vi "current viewer.vi"() -> ()   [LabVIEW 2018]
panel:
  out "Motor Current Versus Time":sgl[][](graph)
  in  "File":path
  # "v1.01"
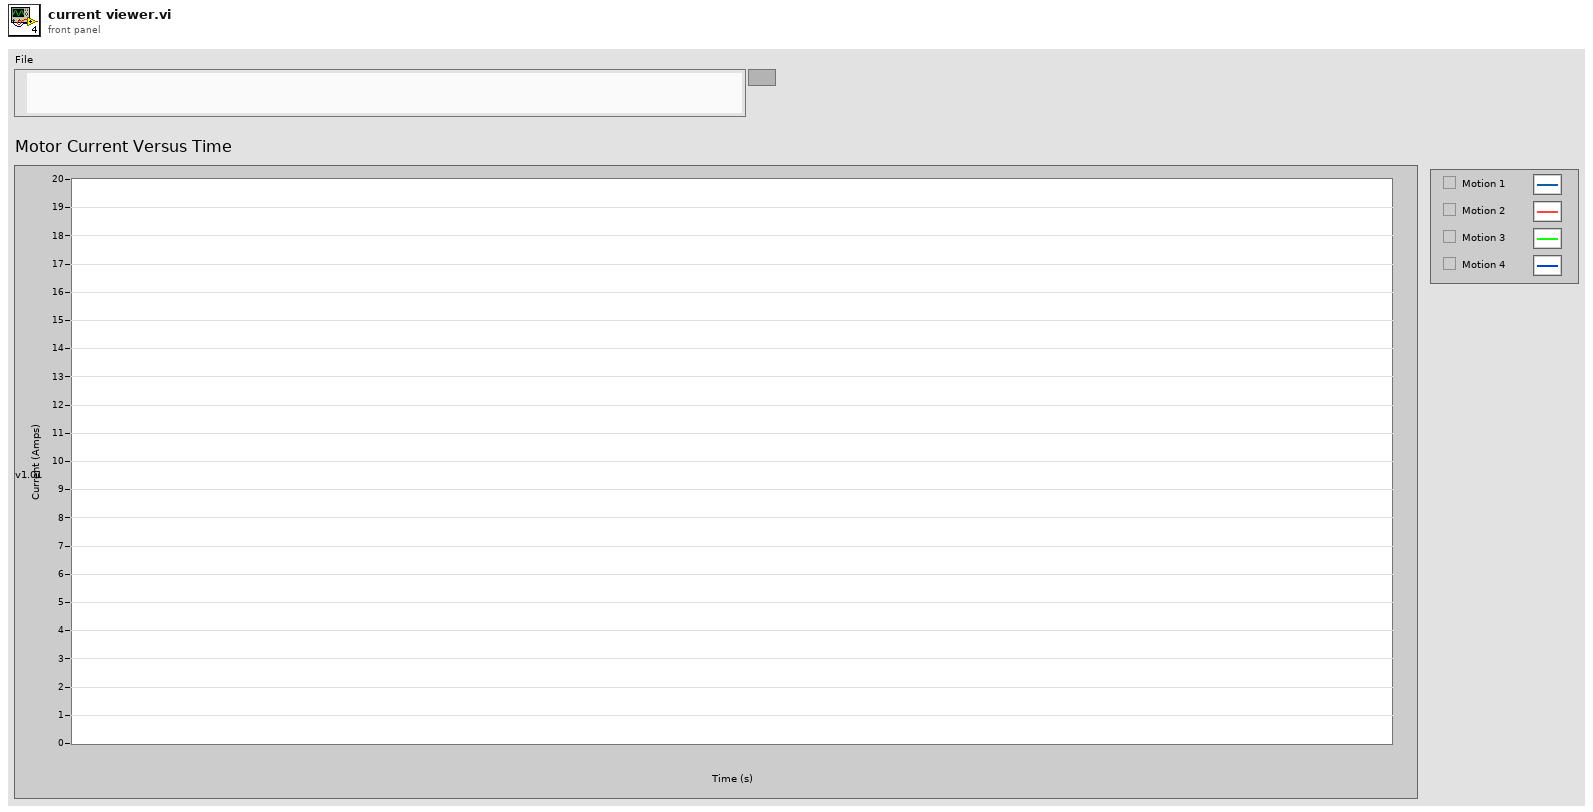
[diagram p1: front panel]
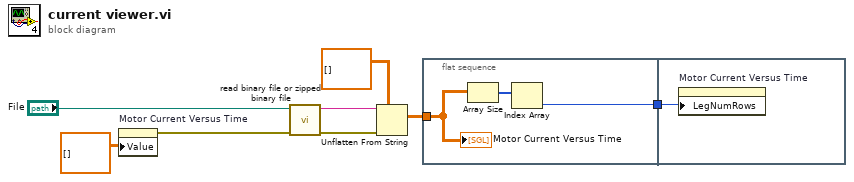
[diagram p0: block diagram]
diagram:
  n1 = property on="Motor Current Versus Time" class="WFGraph (严格)"("Value"=sgl[][] [] ("Motor Current Versus Time")) -> (error out=w6:errorcluster)  [unwired: 2 in, 1 out]
  n2 = call "read binary file or zipped binary file.vi"("error in"=w6, "File"="File") -> ("error out"=w3:errorcluster, "data"=w2:string)  [unwired: 8 in]
  n3 = Unflatten From String(type=sgl[][] [], binary string=w2, error in (no error)=w3) -> (value=w1:sgl[][])  [unwired: 2 in, 2 out]
  n4 = flat-sequence {
    tunnel: w1 -> [w10]
    tunnel: [w9] -> w7
    tunnel: w7 -> [w12]
    frame #0 {
      n5 = Array Size(array=w10) -> (size(s)=w11:i32[])
      n6 = Index Array(array=w11) -> (element=w9:i32)  [unwired: 1 in]
      "Motor Current Versus Time" <- w10
    }
    frame #1 {
      n7 = property on="Motor Current Versus Time" class="WFGraph (严格)"("LegNumRows"=w12) -> ()  [unwired: 2 in, 2 out]
    }
  }
